vi "set_ref_clus_MaxiGauge.vi"(8 "input cluster":T1, 10 "value_array":dbl[](array[numeric])=[0.0, 0.0, 0.0, 0.0, 0.0, 0.0], 11 "status_in":bool) -> ()   [LabVIEW 2019]
uses:
  cluster_ref_MaxiGauge.ctl
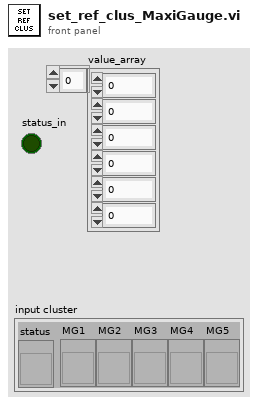
[diagram p1: front panel]
types:
  T1 = typedef "cluster_ref_MaxiGauge.ctl" = cluster{"status":refnum<vi>, "MG1":refnum<vi>, "MG2":refnum<vi>, "MG3":refnum<vi>, "MG4":refnum<vi>, "MG5":refnum<vi>}
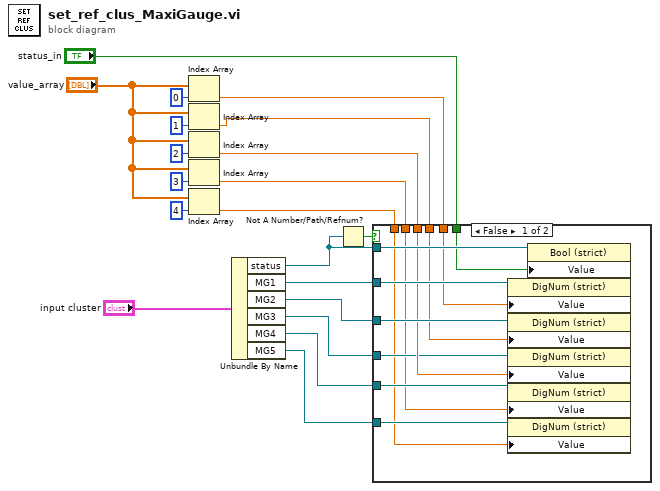
[diagram p0: block diagram]
diagram:
  n1 = Index Array(array="value_array", index=0) -> (element=w12:dbl)
  n2 = Index Array(array="value_array", index=1) -> (element=w8:dbl)
  n3 = Index Array(array="value_array", index=2) -> (element=w7:dbl)
  n4 = Index Array(array="value_array", index=3) -> (element=w6:dbl)
  n5 = Index Array(array="value_array", index=4) -> (element=w2:dbl)
  n6 = Unbundle By Name("input cluster") -> ("status"=w17:refnum<vi>, "MG1"=w18:refnum<vi>, "MG2"=w19:refnum<vi>, "MG3"=w16:refnum<vi>, "MG4"=w14:refnum<vi>, "MG5"=w3:refnum<vi>)
  n7 = Not A Number/Path/Refnum?(number/path/refnum=w17) -> (NaN/Path/Refnum?=w20:bool)
  n8 = case shown="False" w20 {
    tunnel: w18 -> [w32 _]
    tunnel: w19 -> [w31 _]
    tunnel: w17 -> [w30 _]
    tunnel: "status_in" -> [w29 _]
    tunnel: w12 -> [w28 _]
    tunnel: w8 -> [w27 _]
    tunnel: w7 -> [w26 _]
    tunnel: w16 -> [w25 _]
    tunnel: w14 -> [w24 _]
    tunnel: w6 -> [w23 _]
    tunnel: w3 -> [w22 _]
    tunnel: w2 -> [w21 _]
    frame False {
      n9 = property class="DigNum (strict)"(reference=w32, "Value"=w28) -> ()  [unwired: 1 in, 2 out]
      n10 = property class="DigNum (strict)"(reference=w31, "Value"=w27) -> ()  [unwired: 1 in, 2 out]
      n11 = property class="DigNum (strict)"(reference=w25, "Value"=w26) -> ()  [unwired: 1 in, 2 out]
      n12 = property class="DigNum (strict)"(reference=w24, "Value"=w23) -> ()  [unwired: 1 in, 2 out]
      n13 = property class="DigNum (strict)"(reference=w22, "Value"=w21) -> ()  [unwired: 1 in, 2 out]
      n14 = property class="Bool (strict)"(reference=w30, "Value"=w29) -> ()  [unwired: 1 in, 2 out]
    }
    frame True {
    }
  }
